vi "check length and write data to file.vi"(8 "fileIO":T2, 10 "data":variant, 11 "queues":T1) -> (0 "output cluster":T2)   [LabVIEW 2018]
uses:
  type defs/file IO data.ctl
  type defs/channelControl.ctl
  RT/Type Defs/channelScalingTypes.ctl
  RT/Type Defs/scalingMethods.ctl
  Github/ICL-LabVIEW_General/data channels/parent class/Data Channel.lvclass
  type defs/Queues.ctl
  supporting VIs/polymorphic VIs/enqueue for user interface.vi
  supporting VIs/polymorphic VIs/enqueue for file IO.vi
  Github/ICL-LabVIEW_General/data channels/data channels.lvlib
panel:
  out "streaming":bool
  out "points written":u32
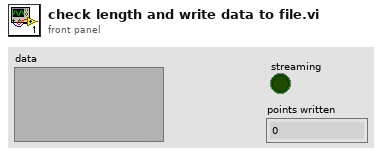
[diagram p1: front panel]
types:
  T1 = typedef "Queues.ctl" = cluster{"messageHandler":refnum<queue>, "comms":refnum<queue>, "dataStream":refnum<queue>, "dataProcessor":refnum<queue>, "fileIO":refnum<queue>, "userInterface":refnum<queue>, "errors":refnum<queue>, "customCompressor":refnum<queue>}
  T2 = typedef "file IO data.ctl" = cluster{"params":cluster{"startFolder":path, "channelConfigPath":path}, "vars":cluster{"channelConfig ":T3[], "writing":cluster{"streaming":bool, "fixedLength":bool, "pointCount":u32, "timeZero":dbl, "pointsWritten":u32, "dataRate":u16}, "channelCount":u16, "fileTarget":cluster{"Save folder":path, "Target filename":string, "file ref":refnum<file>, "pulsatorSpeed":string, "motorSpeed":string, "valvePosition":string, "torqueFilter":bool, "pulsatorRunning":bool, "motorRunning":bool}, "channels":refnum<class "Data Channel.lvclass">[]}}
  T3 = typedef "channelControl.ctl" = cluster{"index":u16, "active":bool, "channelType":T4, "module":u16, "terminal":u16, "channelName":string, "scalingMethod":T5, "scalingParameters":dbl[], "scaledUnits":string, "tempOffset":dbl}
  T4 = typedef "channelScalingTypes.ctl" = enum16{"calculation", "measurement", "scanivalve", "output", "digital"}
  T5 = typedef "scalingMethods.ctl" = enum16{"none", "linear", "thermocouple", "polynomial", "encoder", "RTD"}
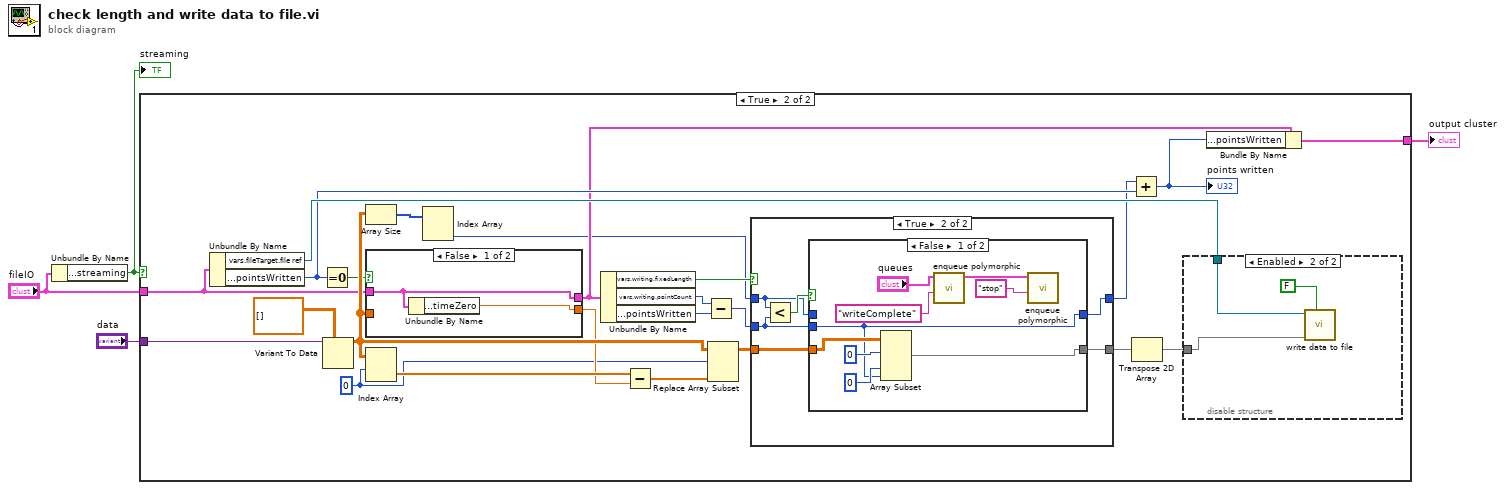
[diagram p0: block diagram]
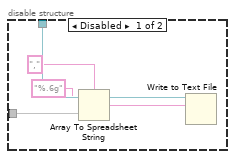
[diagram p3: hidden frame]
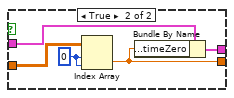
[diagram p6: hidden frame]
diagram:
  n1 = Unbundle By Name("fileIO") -> ("vars.writing.streaming"=w3:bool)
  "streaming" <- w3
  n2 = case shown="True" w3 {
    tunnel: "data" -> [_ w29]
    tunnel: "fileIO" -> [w5 w16]
    tunnel: [w5 w15] -> w1
    frame False {
    }
    frame True {
      w20 = 0 ("index (row)")
      n3 = Unbundle By Name(w16) -> ("vars.fileTarget.file ref"=w26:refnum<file>, "vars.writing.pointsWritten"=w17:u32)
      n4 = Equal To 0?(x=w17) -> (x = 0?=w23:bool)
      n5 = Variant To Data(type=dbl[][] [] ("input 1"), Variant=w29) -> (data=w27:dbl[][])  [unwired: 1 in, 1 out]
      n6 = Array Size(array=w27) -> (size(s)=w25:i32[])
      n7 = case shown="False" w23 {
        tunnel: w27 -> [_ w62]
        tunnel: w16 -> [w57 w61]
        tunnel: [w58 w60] -> w21
        tunnel: [w57 w59] -> w14
        frame False {
          n8 = Unbundle By Name(w57) -> ("vars.writing.timeZero"=w58:dbl)
        }
        frame True {
          w63 = 0 ("index (row)")
          n9 = Index Array(array=w62, index (row)=w63, index (col)=w63) -> (element=w60:dbl)
          n10 = Bundle By Name(cluster=w61, "vars.writing.timeZero"=w60) -> (w59:T2)
        }
      }
      n11 = Index Array(array=w27, index (row)=w20) -> (element=w22:dbl[])  [unwired: 1 in]
      n12 = Index Array(array=w25) -> (element #2=w10:i32)  [unwired: 2 in, 1 out]
      n13 = Unbundle By Name(w14) -> ("vars.writing.fixedLength"=w13:bool, "vars.writing.pointCount"=w8:u32, "vars.writing.pointsWritten"=w7:u32)
      n14 = Subtract(x=w22, y=w21) -> (x-y=w19:dbl[])
      n15 = Subtract(x=w8, y=w7) -> (x-y=w6:u32)
      n16 = Replace Array Subset(array=w27, new element=w19, index (row)=w20) -> (w12:dbl[][])  [unwired: 1 in]
      n17 = case shown="True" w13 {
        tunnel: [w39 w44] -> w11
        tunnel: w12 -> [w39 w43]
        tunnel: w10 -> [w38 w41]
        tunnel: [w38 w42] -> w9
        tunnel: w6 -> [_ w40]
        frame False {
        }
        frame True {
          n18 = Less?(x=w41, y=w40) -> (x < y?=w45:bool)
          n19 = case shown="False" w45 {
            tunnel: [w51 w56] -> w44
            tunnel: w43 -> [w54 w56]
            tunnel: [w50 w55] -> w42
            tunnel: w41 -> [_ w55]
            tunnel: w40 -> [w50 _]
            frame False {
              n20 = Array Subset(array=w54, index (row)=0 ("index"), index (col)=0 ("index"), length (col)=w50) -> (w51:dbl[][])  [unwired: 1 in]
              n21 = call-poly "enqueue polymorphic.vi"("message"="writeComplete", "Queues"="queues") -> ("Queues out"=w47:T1)  [unwired: 9 in]
              n22 = call-poly "enqueue polymorphic.vi"("message"="stop", "Queues"=w47) -> ()  [unwired: 9 in, 1 out]
            }
            frame True {
            }
          }
        }
      }
      n23 = Add(x=w9, y=w17) -> (x+y=w18:u32)
      "points written" <- w18
      n24 = Transpose 2D Array(2D array=w11) -> (transposed array=w24:dbl[][])
      n25 = disable-structure shown="Enabled" {
        disable-tunnel: w26 -> [w34 w36]
        disable-tunnel: w24 -> [w30 w37]
        frame Disabled {
          n26 = Array To Spreadsheet String(delimiter (Tab)=",", array=w30, 3:"%.6g" ("format string")) -> (spreadsheet string=w31:string)
          n27 = Write to Text File(file (use dialog)=w34, text=w31) -> ()  [unwired: 2 in, 3 out]
        }
        frame Enabled {
          n28 = call "write data to file.vi"("useChannelPrecision (T)"=FALSE, "data for writing"=w37, "file reference"=w36) -> ()  [unwired: 7 in, 2 out]
        }
      }
      n29 = Bundle By Name(cluster=w14, "vars.writing.pointsWritten"=w18) -> (w15:T2)
    }
  }
  "output cluster" <- w1
